vi "RSZVB Set Calibration Kit User Connector Type.vi"(8 "error in (no error)":errorcluster {"code" format="%.0x"}, 9 "Calibration Kit Name":string, 10 "Connector":string, 11 "VISA session":refnum<visa-resource-name>) -> (0 "error out":errorcluster {"code" format="%.0x"}, 3 "dup VISA session":refnum<visa-resource-name>)   [LabVIEW 2011]
doc: "This VI selects the calibration kit to be used for a specified connector type.\n\nNote(s):\n\n(1) The VI is suitable for connector types with arbitrary, user-defined names. For standard connector types you can use the command [SENSe<Ch>:]CORRection:CKIT:<conn_type>:SELect (VI rszvb_SetCalibrationKit)\n\nRemote-control command(s):\n[SENSe<Ch>:]CORRection:CKIT:SELect '<conn_name>', '<ckit_name>'"
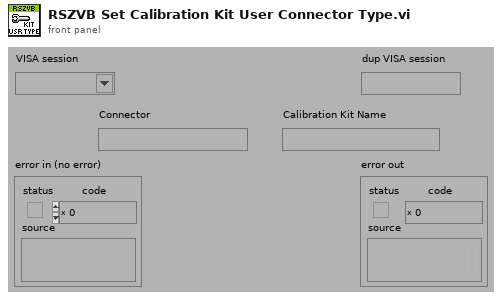
[diagram p1: front panel]
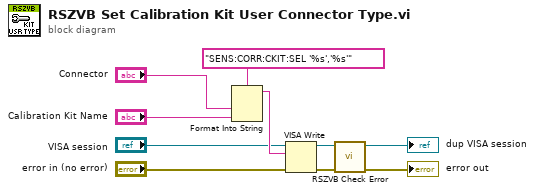
[diagram p0: block diagram]
diagram:
  n1 = Format Into String(format string="SENS:CORR:CKIT:SEL '%s','%s'", "Connector", "Calibration Kit Name") -> (resulting string=w7:string)  [unwired: 2 in, 1 out]
  n2 = VISA Write(VISA resource name="VISA session", write buffer=w7, error in (no error)="error in (no error)") -> (VISA resource name out=w9:refnum<visa-resource-name>, error out=w10:errorcluster)  [unwired: 1 out]
  n3 = call "RSZVB Check Error.vi"("error in (no error)"=w10, "VISA session"=w9) -> ("error out"=→"error out":errorcluster, "dup VISA session"=→"dup VISA session":refnum<visa-resource-name>)  [unwired: 8 in]
